vi "Check if same stim and Imaging Path.vi"(11 "System Information Cluster":T1) -> (3 "Boolean":bool)   [LabVIEW 2012]
uses:
  Custom Controls and Typedefs/SciScan System Information Cluster.ctl
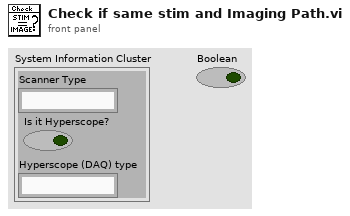
[diagram p1: front panel]
types:
  T1 = typedef "SciScan System Information Cluster.ctl" = cluster{"Scanner Type":string, "Is it Hyperscope?":bool, "Hyperscope (DAQ) type":string}
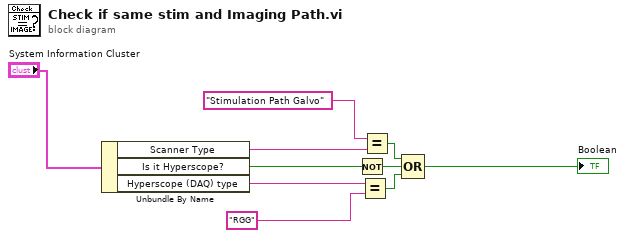
[diagram p0: block diagram]
diagram:
  n1 = Unbundle By Name("System Information Cluster") -> ("Scanner Type"=w8:string, "Is it Hyperscope?"=w7:bool, "Hyperscope (DAQ) type"=w6:string)
  n2 = Not(x=w7) -> (.not. x?=w3:bool)
  n3 = Equal?(x=w6, y="RGG") -> (x = y?=w4:bool)
  n4 = Equal?(x="Stimulation Path Galvo", y=w8) -> (x = y?=w2:bool)
  n5 = Compound Arithmetic op=OR(w2, w3, w4) -> (→"Boolean":bool)
